vi "Init.vi"(8 "error in (no error)":errorcluster, 9 "Constant Action Data":string, 10 "HAL GOOP4.lvlib:Instrument Base":refnum<class "Instrument.lvclass">, 11 "Virt Instrument Base in":refnum<class "Virt Waveform Reader.lvclass">) -> (0 "error out":errorcluster, 3 "Virt Instrument Base out":refnum<class "Virt Waveform Reader.lvclass">)   [LabVIEW 2023, in "Virt Instrs Scope.lvlib" / "Virt Waveform Reader.lvclass"]
uses:
  Virt Waveform Reader.lvclass
  Instrument/Instrument.lvclass
  Virtual Instrument Base/Virt Instr Base.lvclass
  Virt Waveform Reader.lvclass/Virt Waveform Reader.ctl
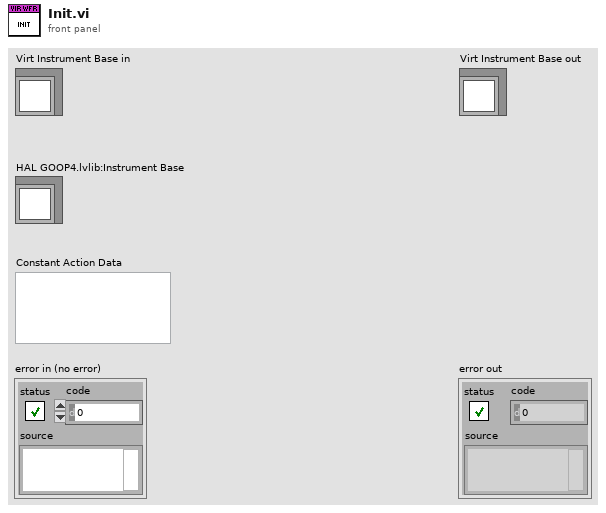
[diagram p1: front panel]
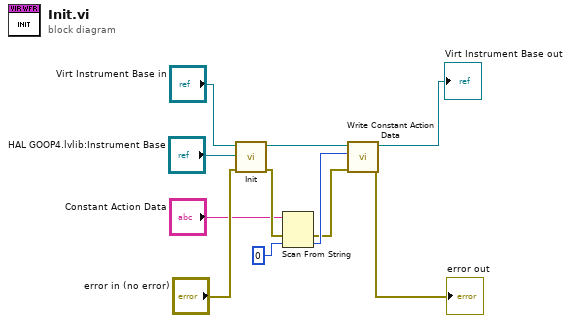
[diagram p0: block diagram]
diagram:
  n1 = call-parent "Init.vi"("error in (no error)"="error in (no error)", "HAL GOOP4.lvlib:Instrument"="HAL GOOP4.lvlib:Instrument Base", "Virt Instrument Base in"="Virt Instrument Base in") -> ("error out"=w5:errorcluster, "Virt Instrument Base out"=w7:refnum<class "Virt Waveform Reader.lvclass">)  [unwired: 7 in]
  n2 = Scan From String(input string="Constant Action Data", error in=w5, default 1=u8 0) -> (error out=w2:errorcluster, output 1=w3:u8)  [unwired: 2 in, 2 out]
  n3 = call "Write Constant Action Data.vi"("error in (no error)"=w2, "Constant Action Data"=w3, "Virt Instrument Base in"=w7) -> ("error out"=→"error out":errorcluster, "Virt Instrument Base out"=→"Virt Instrument Base out":refnum<class "Virt Waveform Reader.lvclass">)  [unwired: 7 in]
